vi "Get Versions from COM Devices.vi"(0 "port":refnum<visa-resource-name>, 11 "error in (no error)":errorcluster) -> (4 "port out":refnum<visa-resource-name>, 8 "versions":T1, 15 "error out":errorcluster)   [LabVIEW 2010]
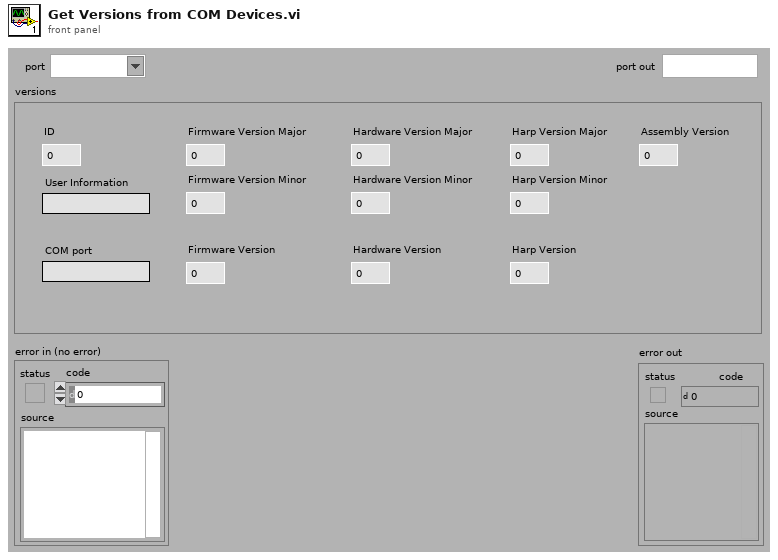
[diagram p1: front panel]
types:
  T1 = cluster{"Firmware Version Major":u8, "Firmware Version Minor":u8, "Hardware Version Major":u8, "Hardware Version Minor":u8, "Harp Version Major":u8, "Harp Version Minor":u8, "Assembly Version":u8, "Firmware Version":dbl, "Hardware Version":dbl, "Harp Version":dbl, "ID":u16, "User Information":string, "COM port":string}
  T2 = cluster{"Firmware Version Major":u8, "Firmware Version Minor":u8, "Hardware Version Major":u8, "Hardware Version Minor":u8, "Harp Version Major":u8, "Harp Version Minor":u8, "Assembly Version":u8, "Firmware Version":dbl, "Hardware Version":dbl, "Harp Version":dbl, "ID":u16, "User Information":string, "COM ports":string}
  T3 = cluster{"Timestamp(us)":dbl, "Command":u8, "Error":bool, "Register Address":u8, "Port":u8, "Number of Elements":u8, "Type":u8, "I8":i8, "U8":u8, "U16":u16, "I16":i16, "U32":u32, "I32":i32, "U64":u64, "I64":i64, "Float":sgl, "U8[]":u8[], "I8[]":i8[], "U16[]":u16[], "I16[]":i16[], "U32[]":u32[], "I32[]":i32[], "U64[]":u64[], "I64[]":i64[], "Float[]":sgl[]}
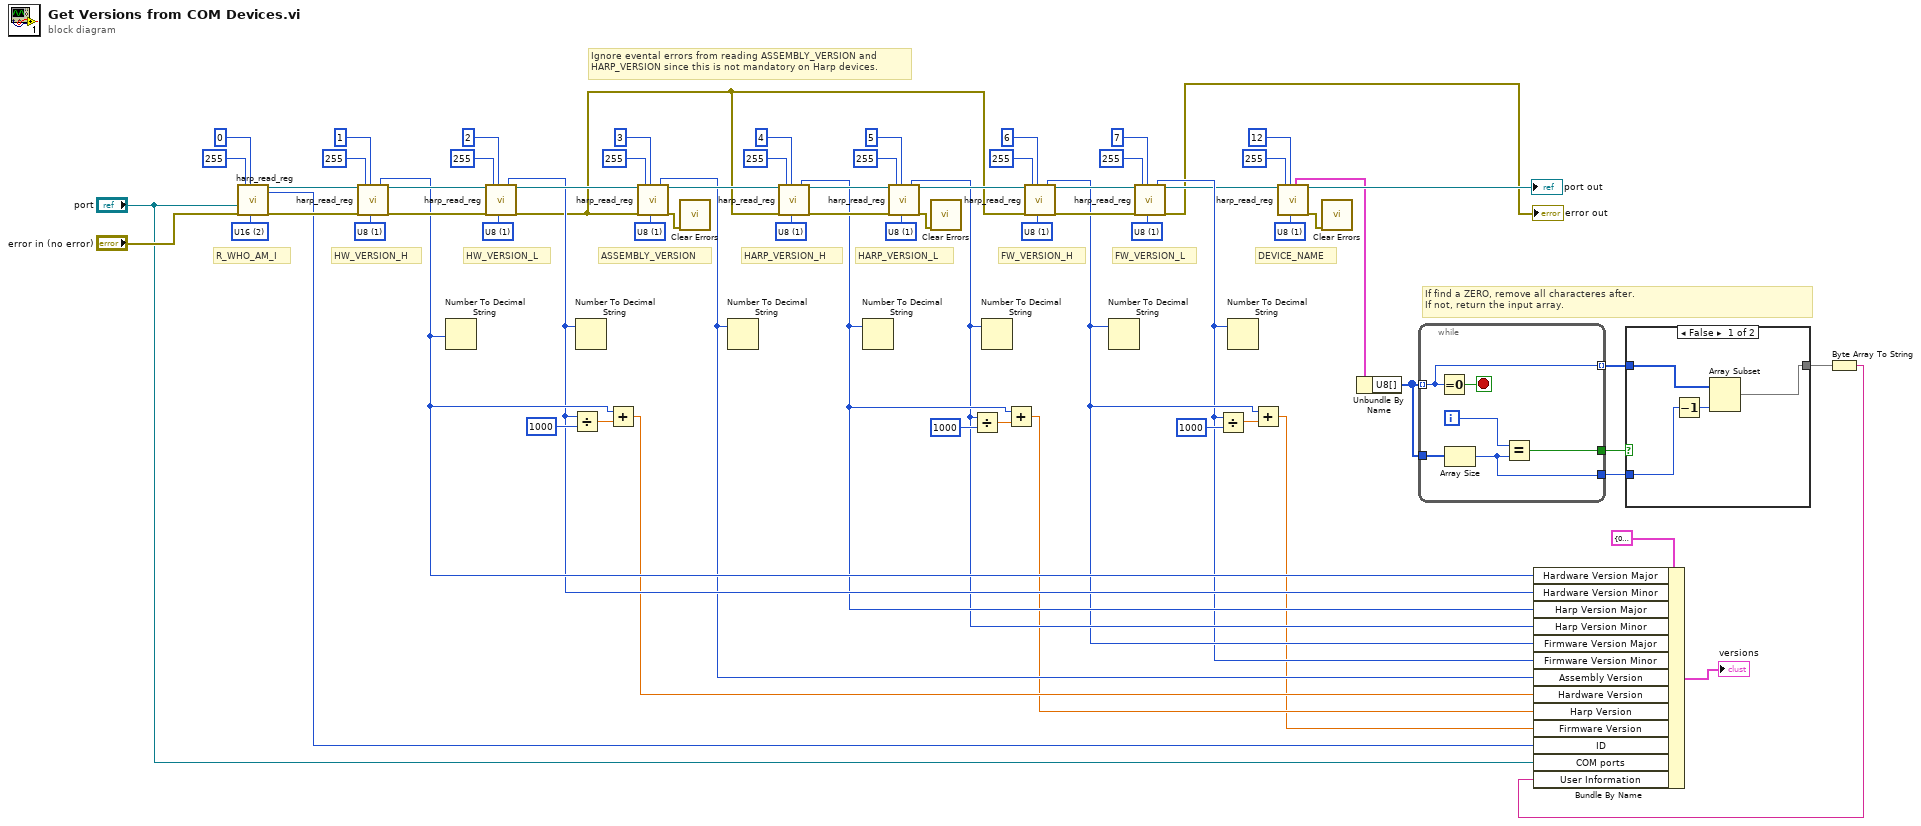
[diagram p0: block diagram]
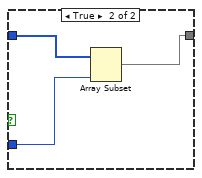
[diagram p2: hidden frame]
diagram:
  w15 = u8 1 items=["U8"=1, "U16"=2, "U32"=4, "U64"=8, "I8"=129, "I16"=130, "I32"=132, "I64"=136, "FLOAT"=68, "BOOL"=17] ("type")
  w45 = u8 1 items=["U8"=1, "U16"=2, "U32"=4, "U64"=8, "I8"=129, "I16"=130, "I32"=132, "I64"=136, "FLOAT"=68, "BOOL"=17] ("type")
  w52 = u8 1 items=["U8"=1, "U16"=2, "U32"=4, "U64"=8, "I8"=129, "I16"=130, "I32"=132, "I64"=136, "FLOAT"=68, "BOOL"=17] ("type")
  w53 = u8 1 items=["U8"=1, "U16"=2, "U32"=4, "U64"=8, "I8"=129, "I16"=130, "I32"=132, "I64"=136, "FLOAT"=68, "BOOL"=17] ("type")
  w60 = u8 1 items=["U8"=1, "U16"=2, "U32"=4, "U64"=8, "I8"=129, "I16"=130, "I32"=132, "I64"=136, "FLOAT"=68, "BOOL"=17] ("type")
  w59 = u8 1 items=["U8"=1, "U16"=2, "U32"=4, "U64"=8, "I8"=129, "I16"=130, "I32"=132, "I64"=136, "FLOAT"=68, "BOOL"=17] ("type")
  w67 = u8 1 items=["U8"=1, "U16"=2, "U32"=4, "U64"=8, "I8"=129, "I16"=130, "I32"=132, "I64"=136, "FLOAT"=68, "BOOL"=17] ("type")
  w68 = u8 1 items=["U8"=1, "U16"=2, "U32"=4, "U64"=8, "I8"=129, "I16"=130, "I32"=132, "I64"=136, "FLOAT"=68, "BOOL"=17] ("type")
  w73 = u8 2 items=["U8"=1, "U16"=2, "U32"=4, "U64"=8, "I8"=129, "I16"=130, "I32"=132, "I64"=136, "FLOAT"=68, "BOOL"=17] ("type")
  # "Ignore evental errors from reading ASSEMBLY_VERSION and\nHARP_VERSION since this is not mandatory on Harp devices."
  # "If find a ZERO, remove all characteres after.\nIf not, return the input array."
  # "DEVICE_NAME"
  # "HW_VERSION_L"
  # "FW_VERSION_L"
  # "FW_VERSION_H"
  # "HARP_VERSION_L"
  # "HARP_VERSION_H"
  # "ASSEMBLY_VERSION"
  # "HW_VERSION_H"
  # "R_WHO_AM_I"
  n1 = call "harp_read_reg.vi"(0:"port"="port", "error in (no error)"="error in (no error)", 6:"port"=u8 255 ("port"), "reg. address"=u8 0, "type"=w73) -> ("port out"=w39:refnum<visa-resource-name>, "16 bits"=w22:u16, "error out"=w40:errorcluster)  [unwired: 5 in, 7 out]
  n2 = call "harp_read_reg.vi"(0:"port"=w39, "error in (no error)"=w40, 6:"port"=u8 255 ("port"), "reg. address"=u8 1, "type"=w68) -> ("8 bits"=w32:u8, "port out"=w43:refnum<visa-resource-name>, "error out"=w44:errorcluster)  [unwired: 5 in, 7 out]
  n3 = Number To Decimal String(number=w32) -> ()  [unwired: 1 in, 1 out]
  n4 = call "harp_read_reg.vi"(0:"port"=w43, "error in (no error)"=w44, 6:"port"=u8 255 ("port"), "reg. address"=u8 2, "type"=w45) -> ("8 bits"=w31:u8, "port out"=w42:refnum<visa-resource-name>, "error out"=w3:errorcluster)  [unwired: 5 in, 7 out]
  n5 = Divide(x=w31, y=u32 1000) -> (x/y=w35:dbl)
  n6 = Number To Decimal String(number=w31) -> ()  [unwired: 1 in, 1 out]
  n7 = Add(x=w32, y=w35) -> (x+y=w25:dbl)
  n8 = call "harp_read_reg.vi"(0:"port"=w42, "error in (no error)"=w3, 6:"port"=u8 255 ("port"), "reg. address"=u8 3, "type"=w67) -> ("8 bits"=w26:u8, "port out"=w56:refnum<visa-resource-name>, "error out"=w2:errorcluster)  [unwired: 5 in, 7 out]
  n9 = call <vilib>:"Clear Errors.vi"("error in (no error)"=w2) -> ()  [unwired: 6 in, 1 out]
  n10 = Number To Decimal String(number=w26) -> ()  [unwired: 1 in, 1 out]
  n11 = call "harp_read_reg.vi"(0:"port"=w56, "error in (no error)"=w3, 6:"port"=u8 255 ("port"), "reg. address"=u8 4, "type"=w59) -> ("8 bits"=w30:u8, "port out"=w63:refnum<visa-resource-name>, "error out"=w64:errorcluster)  [unwired: 5 in, 7 out]
  n12 = Number To Decimal String(number=w30) -> ()  [unwired: 1 in, 1 out]
  n13 = call "harp_read_reg.vi"(0:"port"=w63, "error in (no error)"=w64, 6:"port"=u8 255 ("port"), "reg. address"=u8 5, "type"=w60) -> ("8 bits"=w29:u8, "port out"=w47:refnum<visa-resource-name>, "error out"=w1:errorcluster)  [unwired: 5 in, 7 out]
  n14 = call <vilib>:"Clear Errors.vi"("error in (no error)"=w1) -> ()  [unwired: 6 in, 1 out]
  n15 = Divide(x=w29, y=u32 1000) -> (x/y=w34:dbl)
  n16 = Number To Decimal String(number=w29) -> ()  [unwired: 1 in, 1 out]
  n17 = Add(x=w30, y=w34) -> (x+y=w24:dbl)
  n18 = call "harp_read_reg.vi"(0:"port"=w47, "error in (no error)"=w3, 6:"port"=u8 255 ("port"), "reg. address"=u8 6, "type"=w53) -> ("8 bits"=w28:u8, "port out"=w49:refnum<visa-resource-name>, "error out"=w48:errorcluster)  [unwired: 5 in, 7 out]
  n19 = Number To Decimal String(number=w28) -> ()  [unwired: 1 in, 1 out]
  n20 = call "harp_read_reg.vi"(0:"port"=w49, "error in (no error)"=w48, 6:"port"=u8 255 ("port"), "reg. address"=u8 7, "type"=w52) -> ("8 bits"=w27:u8, "port out"=w14:refnum<visa-resource-name>, "error out"=→"error out":errorcluster)  [unwired: 5 in, 7 out]
  n21 = Divide(x=w27, y=u32 1000) -> (x/y=w33:dbl)
  n22 = Number To Decimal String(number=w27) -> ()  [unwired: 1 in, 1 out]
  n23 = Add(x=w28, y=w33) -> (x+y=w23:dbl)
  n24 = call "harp_read_reg.vi"(0:"port"=w14, 6:"port"=u8 255 ("port"), "reg. address"=u8 12, "type"=w15) -> ("HarpDataFrame"=w12:T3, "port out"=→"port out":refnum<visa-resource-name>, "error out"=w4:errorcluster)  [unwired: 6 in, 7 out]
  n25 = call <vilib>:"Clear Errors.vi"("error in (no error)"=w4) -> ()  [unwired: 6 in, 1 out]
  n26 = Unbundle By Name(w12) -> ("U8[]"=w8:u8[])
  n27 = while {
    tunnel: w8 -> [w78] mode=indexing
    tunnel: [w78] -> w10 mode=indexing
    tunnel: w8 -> [w77]
    tunnel: [w75] -> w11
    tunnel: [w74] -> w9
    i -> [w76]
    stop <- w79 stop-if-true
    n28 = Equal To 0?(x=w78) -> (x = 0?=w79:bool)
    n29 = Array Size(array=w77) -> (size(s)=w74:i32)
    n30 = Equal?(x=w76, y=w74) -> (x = y?=w75:bool)
  }
  n31 = case shown="False" w11 {
    tunnel: [w80 w85] -> w7
    tunnel: w10 -> [w81 w86]
    tunnel: w9 -> [w82 w84]
    frame False {
      n32 = Decrement(x=w82) -> (x-1=w83:i32)
      n33 = Array Subset(array=w81, length=w83) -> (w80:u8[])  [unwired: 1 in]
    }
    frame True {
      n34 = Array Subset(array=w86, length=w84) -> (w85:u8[])  [unwired: 1 in]
    }
  }
  n35 = Byte Array To String(unsigned byte array=w7) -> (string=w6:string)
  n36 = Bundle By Name(cluster=T2 {"Firmware Version Major"=0, "Firmware Version Minor"=0, "Hardware Version Major"=0, "Hardware Version Minor"=0, "Harp Version Major"=0, "Harp Version Minor"=0, "Assembly Version"=0, "Firmware Version"=0.0, "Hardware Version"=0.0, "Harp Version"=0.0, "ID"=0, "User Information"="", "COM ports"=""} ("versions"), "Hardware Version Major"=w32, "Hardware Version Minor"=w31, "Harp Version Major"=w30, "Harp Version Minor"=w29, "Firmware Version Major"=w28, "Firmware Version Minor"=w27, "Assembly Version"=w26, "Hardware Version"=w25, "Harp Version"=w24, "Firmware Version"=w23, "ID"=w22, "COM ports"="port", "User Information"=w6) -> (→"versions":T2)
